vi "DeleteMemory.vi"(2 "error in (no error)":errorcluster, 3 "Configuration Name":string, 4 "Delete Memory / Configuration":u16(ring) items=["Memory 0", "Memory 1", "Memory 2", "Memory 3", "Memory 4", "Configuration"], 5 "VISA resource name":refnum<visa-resource-name>) -> (0 "error out":errorcluster, 1 "VISA resource name out":refnum<visa-resource-name>)   [LabVIEW 2020, in "Active Technologies AWG3000.lvlib"]
uses:
  Active Technologies AWG3000.lvlib
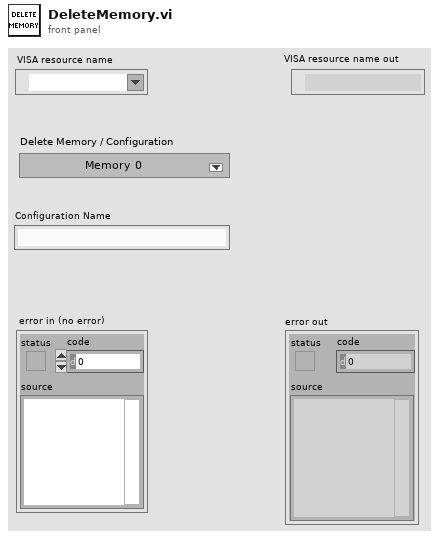
[diagram p1: front panel]
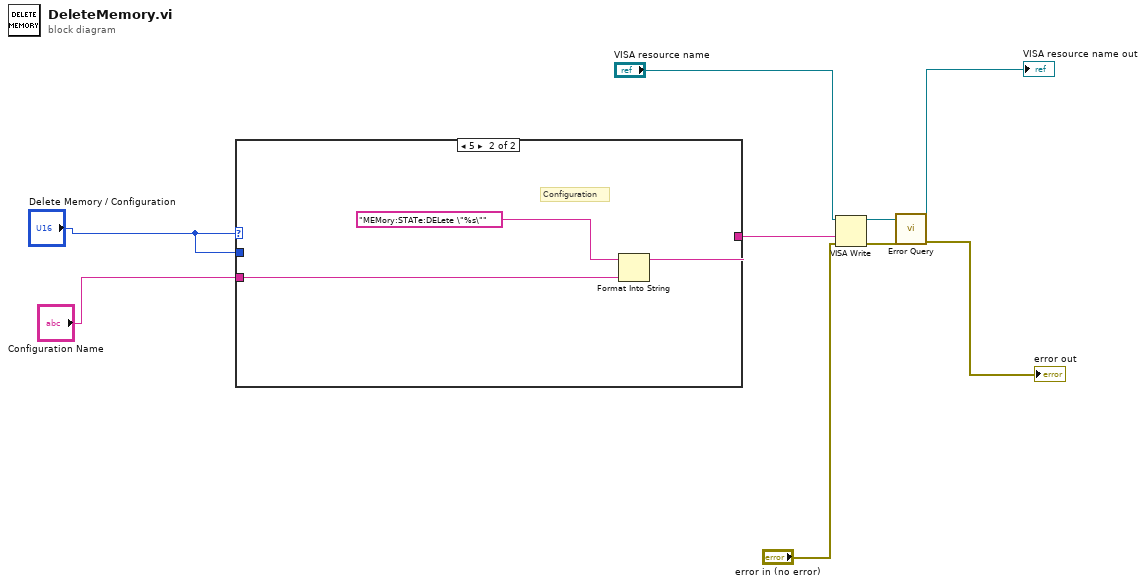
[diagram p0: block diagram]
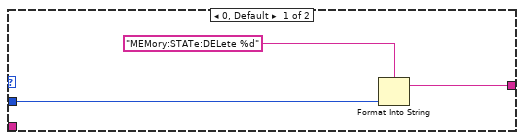
[diagram p2: hidden frame]
diagram:
  n1 = case shown="5" "Delete Memory / Configuration" {
    tunnel: [w11 w13] -> w7
    tunnel: "Delete Memory / Configuration" -> [w10 _]
    tunnel: "Configuration Name" -> [_ w14]
    frame 0, Default {
      n2 = Format Into String(format string="MEMory:STATe:DELete %d" ("write buffer"), w10) -> (resulting string=w11:string)  [unwired: 2 in, 1 out]
    }
    frame 5 {
      # "Configuration"
      n3 = Format Into String(format string="MEMory:STATe:DELete \"%s\"" ("write buffer"), w14) -> (resulting string=w13:string)  [unwired: 2 in, 1 out]
    }
  }
  n4 = VISA Write(VISA resource name="VISA resource name", write buffer=w7, error in (no error)="error in (no error)") -> (VISA resource name out=w6:refnum<visa-resource-name>, error out=w5:errorcluster)  [unwired: 1 out]
  n5 = call "Error Query.vi"("error in (no error)"=w5, "VISA resource name"=w6) -> ("error out"=→"error out":errorcluster, "VISA resource name out"=→"VISA resource name out":refnum<visa-resource-name>)  [unwired: 6 in, 2 out]
